vi "Apply Schedule Core.vi"(8 "error in (no error)":errorcluster, 9 "Settings":variant, 10 "Schedule":u16(ring) items=["Constant", "Ramp", "Function", "Formula"], 11 "Tool Object in":refnum<class "Tool Object.lvclass">) -> (0 "error out":errorcluster, 2 "Schedule Array":dbl[](array[numeric]), 3 "Tool Object out":refnum<class "Tool Object.lvclass">)   [LabVIEW 2019, in "Tool Object.lvclass"]
uses:
  Tool Object.lvclass
  subVIs/typedefs/Schedule - enum.ctl
  subVIs/typedefs/Schedule Types/Schedule--Constant.ctl
  subVIs/typedefs/Schedule Types/Schedule--Ramp.ctl
  subVIs/typedefs/Schedule Types/Schedule--Function Generator.ctl
  subVIs/typedefs/Schedule Types/Schedule--Formula.ctl
  <vilib>/Analysis/1siggen.llb/Ramp Pattern by Samples.vi
  Settings/ObjectSettings/ObjectSettings.lvclass
  <vilib>/Analysis/NI_AALBase.lvlib
  <vilib>/measure/NI_MABase.lvlib
  <vilib>/gmath/NI_Gmath.lvlib
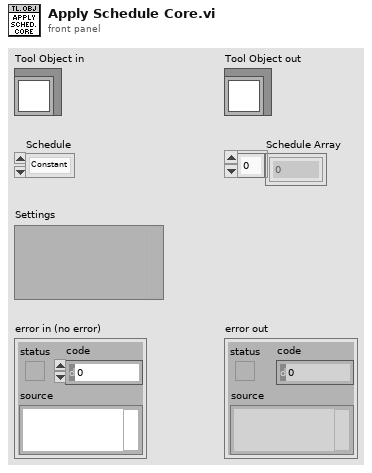
[diagram p1: front panel]
types:
  T1 = typedef "Schedule - enum.ctl" = enum16{"Constant", "Ramp", "Fn. Generator", "Formula"}
  T2 = typedef "PathCommands.lvclass/Point.ctl" = cluster{"X":dbl, "Y":dbl}
  T3 = enum16{"Sine Wave", "Triangle Wave", "Square Wave", "Sawtooth Wave"}
  T4 = typedef "Schedule--Constant.ctl" = cluster{"Value":dbl}
  T5 = typedef "Schedule--Ramp.ctl" = cluster{"Start":dbl, "End":dbl}
  T6 = typedef "Schedule--Function Generator.ctl" = cluster{"Min Value":dbl, "Max Value":dbl, "Duty Cycle (%)":dbl, "Signal Type":u16, "Cycle Number":dbl, "Phase (degrees)":dbl}
  T7 = typedef "Schedule--Formula.ctl" = cluster{"formula":string, "formula length (nm)":dbl, "formula resolution (nm)":dbl}
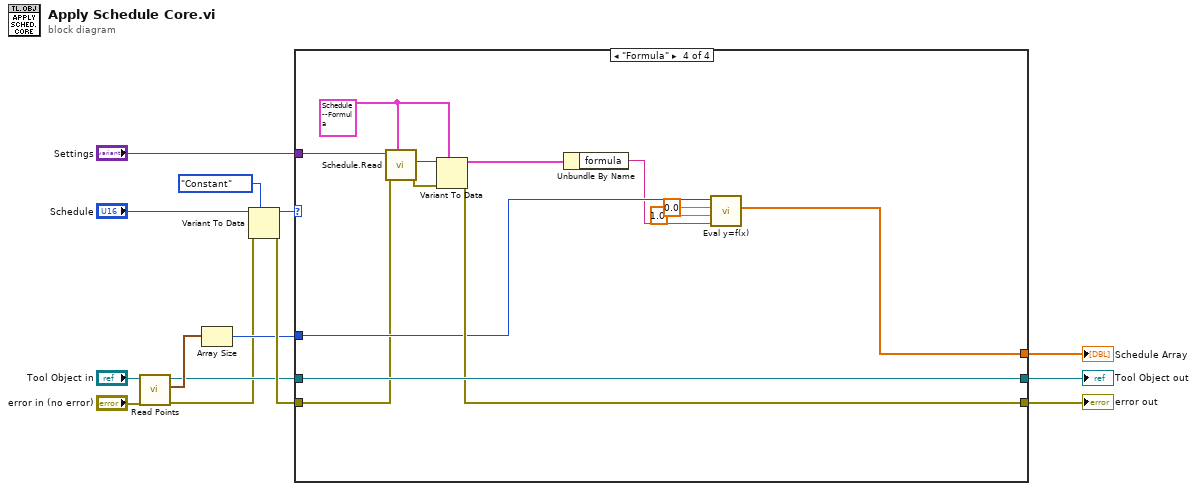
[diagram p0: block diagram]
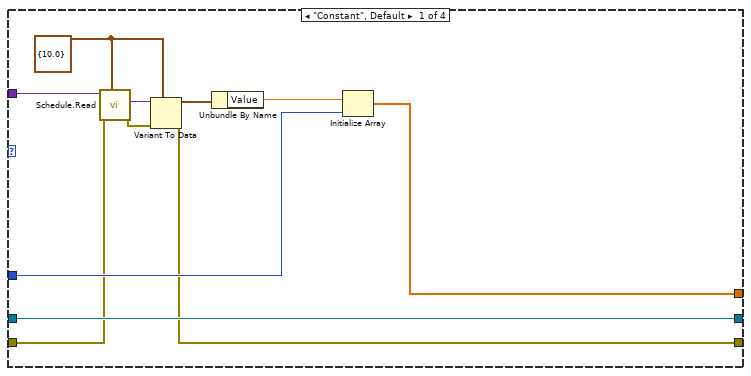
[diagram p2: hidden frame]
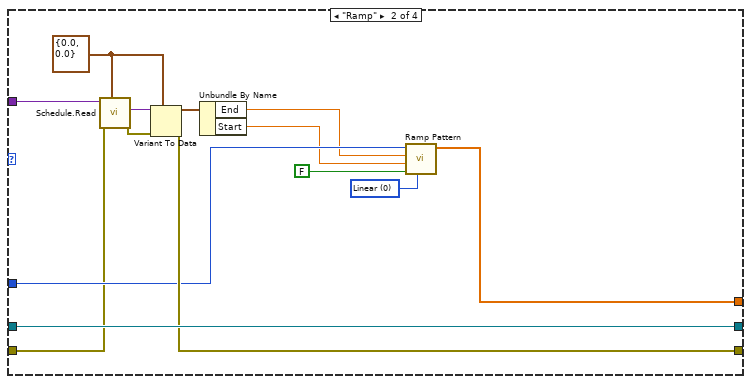
[diagram p3: hidden frame]
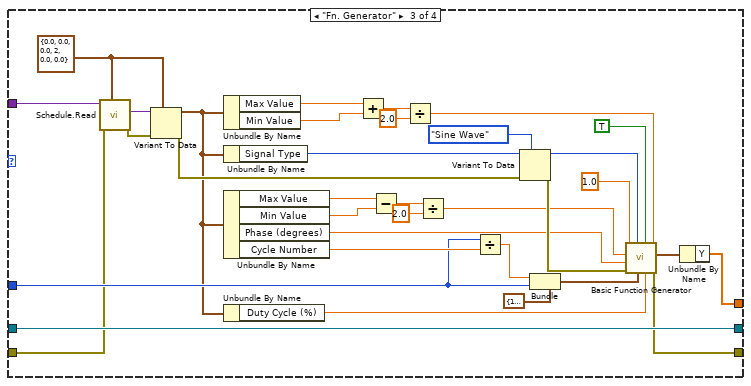
[diagram p4: hidden frame]
diagram:
  n1 = call-dynamic "Read Points.vi"("error in (no error)"="error in (no error)", "Tool Object in"="Tool Object in") -> ("error out"=w1:errorcluster, "Points"=w11:T2[], "Tool Object out"=w6:refnum<class "Tool Object.lvclass">)  [unwired: 7 in]
  n2 = Array Size(array=w11) -> (size(s)=w10:i32)
  n3 = Variant To Data(error in=w1, type=Schedule_-_enum."Constant" ("Schedule"), Variant="Schedule") -> (data=w13:T1, error out=w12:errorcluster)
  n4 = case shown="\"Formula\"" w13 {
    tunnel: w6 -> [w25 w39 w73 w86]
    tunnel: [w25 w39 w73 w86] -> w4
    tunnel: w12 -> [w15 w26 w40 w74]
    tunnel: [w17 w37 w49 w81] -> w5
    tunnel: w10 -> [w19 w35 w50 w78]
    tunnel: [w18 w30 w43 w77] -> w9
    tunnel: "Settings" -> [w16 w27 w41 w75]
    frame "Constant", Default {
      w22 = T4 {"Value"=10.0} ("Constant")
      n5 = call "Schedule.Read.vi"("Data to Read"=w22, "error in (no error)"=w15, "LUT In"=w16) -> ("error out"=w23:errorcluster, "Data Out"=w24:variant)  [unwired: 6 in, 1 out]
      n6 = Variant To Data(error in=w23, type=w22, Variant=w24) -> (data=w21:T4, error out=w17:errorcluster)
      n7 = Unbundle By Name(w21) -> ("Value"=w20:dbl)
      n8 = Initialize Array(w20, w19) -> (w18:dbl[])
    }
    frame "Ramp" {
      w34 = u16 0 items=["Linear", "Logarithmic"] ("type")
      w36 = T5 {"Start"=0.0, "End"=0.0} ("Ramp")
      n9 = call "Schedule.Read.vi"("Data to Read"=w36, "error in (no error)"=w26, "LUT In"=w27) -> ("error out"=w28:errorcluster, "Data Out"=w38:variant)  [unwired: 6 in, 1 out]
      n10 = Variant To Data(error in=w28, type=w36, Variant=w38) -> (data=w33:T5, error out=w37:errorcluster)
      n11 = Unbundle By Name(w33) -> ("End"=w29:dbl, "Start"=w32:dbl)
      n12 = call-poly <vilib>:"Ramp Pattern.vi"("type"=w34, "exclude end?"=FALSE, "start"=w32, "end"=w29, "samples"=w35) -> ("Ramp Pattern"=w30:dbl[])  [unwired: 5 in, 1 out]
    }
    frame "Fn. Generator" {
      w70 = T6 {"Min Value"=0.0, "Max Value"=0.0, "Duty Cycle (%)"=0.0, "Signal Type"=2, "Cycle Number"=0.0, "Phase (degrees)"=0.0} ("Fn. Gen")
      n13 = call "Schedule.Read.vi"("Data to Read"=w70, "error in (no error)"=w40, "LUT In"=w41) -> ("error out"=w72:errorcluster, "Data Out"=w71:variant)  [unwired: 6 in, 1 out]
      n14 = Variant To Data(error in=w72, type=w70, Variant=w71) -> (data=w44:T6, error out=w47:errorcluster)
      n15 = Unbundle By Name(w44) -> ("Max Value"=w51:dbl, "Min Value"=w52:dbl)
      n16 = Unbundle By Name(w44) -> ("Signal Type"=w61:u16)
      n17 = Unbundle By Name(w44) -> ("Max Value"=w57:dbl, "Min Value"=w58:dbl, "Phase (degrees)"=w46:dbl, "Cycle Number"=w65:dbl)
      n18 = Unbundle By Name(w44) -> ("Duty Cycle (%)"=w69:dbl)
      n19 = Add(x=w51, y=w52) -> (x+y=w53:dbl)
      n20 = Subtract(x=w57, y=w58) -> (x-y=w56:dbl)
      n21 = Divide(x=w53, y=2.0) -> (x/y=w59:dbl)
      n22 = Divide(x=w56, y=2.0) -> (x/y=w45:dbl)
      n23 = Divide(x=w50, y=w65) -> (x/y=w67:dbl)
      n24 = Variant To Data(error in=w47, type=T3."Sine Wave" ("signal type"), Variant=w61) -> (data=w63:T3, error out=w48:errorcluster)
      n25 = Bundle(cluster=cluster{"Fs":dbl, "#s":dbl} {"Fs"=1000.0, "#s"=1000.0} ("sampling info"), "Fs"=w67, "#s"=w50) -> (w68:cluster{"Fs":dbl, "#s":dbl})
      n26 = call <vilib>:"Basic Function Generator.vi"("offset"=w59, "square wave duty cycle (%)"=w69, "reset signal"=TRUE, "sampling info"=w68, "signal type"=w63, "error in (no error)"=w48, "phase"=w46, "amplitude"=w45, "frequency"=1.0) -> ("error out"=w49:errorcluster, "signal out"=w42:waveform(dbl))  [unwired: 1 out]
      n27 = Unbundle By Name(w42) -> ("Y"=w43:dbl[])
    }
    frame "Formula" {
      w84 = T7 {"formula"="1*(step(170-t)*cos(0.62831853071*t)+step(t-170)*cos(0.62831853071*(t-170))*(-1))", "formula length (nm)"=340.0, "formula resolution (nm)"=0.001} ("Formula")
      n28 = call "Schedule.Read.vi"("Data to Read"=w84, "error in (no error)"=w74, "LUT In"=w75) -> ("error out"=w85:errorcluster, "Data Out"=w83:variant)  [unwired: 6 in, 1 out]
      n29 = Variant To Data(error in=w85, type=w84, Variant=w83) -> (data=w82:T7, error out=w81:errorcluster)
      n30 = Unbundle By Name(w82) -> ("formula"=w76:string)
      n31 = call <vilib>:"Eval y=f(x).vi"("formula"=w76, "end"=1.0, "start"=0.0, "number of points"=w78) -> ("Y Values"=w77:dbl[])  [unwired: 3 out]
    }
  }
  "error out" <- w5
  "Tool Object out" <- w4
  "Schedule Array" <- w9
